vi "Hide WND.vi"(0 "hwnd":u32, 11 "error in (no error)":errorcluster) -> (15 "error out":errorcluster)   [LabVIEW 2016, in "Py Doc.lvclass"]
uses:
  Py Doc.lvclass
  user32.dll
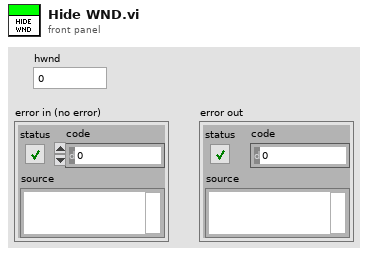
[diagram p1: front panel]
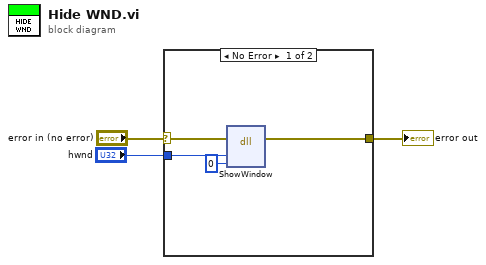
[diagram p0: block diagram]
diagram:
  n1 = case shown="No Error" "error in (no error)" {
    selector: "error in (no error)" -> [w5 w8]
    tunnel: "hwnd" -> [w7 _]
    tunnel: [w6 w8] -> w2
    frame No Error {
      n2 = dll-call lib="user32.dll" fn="ShowWindow"(error in=w5, "hwnd"=w7, "nCmdShow"=u32 0) -> (error out=w6:errorcluster)  [unwired: 5 in, 1 out]
    }
    frame Error {
    }
  }
  "error out" <- w2
